vi "Abbreviate TDMS Group Channel.vi"(9 "Channel":string, 10 "Group":string, 11 "File Path Control":path) -> (2 "Cluster":T1, 3 "Abbreviated":string)   [LabVIEW 2019]
uses:
  File_Group_Chan_Abbr.ctl
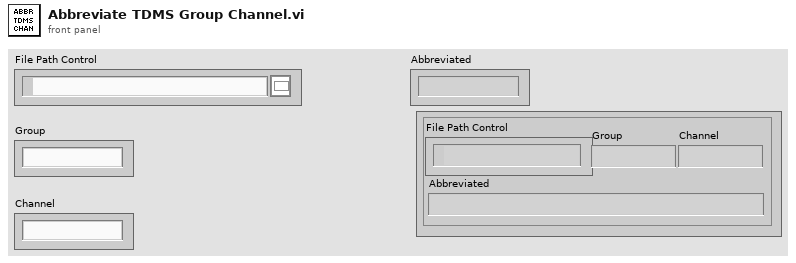
[diagram p1: front panel]
types:
  T1 = typedef "File_Group_Chan_Abbr.ctl" = cluster{"File Path Control":path, "Group":string, "Channel":string, "Abbreviated":string}
  T2 = cluster{"File Path Control":path, "Group":string, "Channel":string, string}
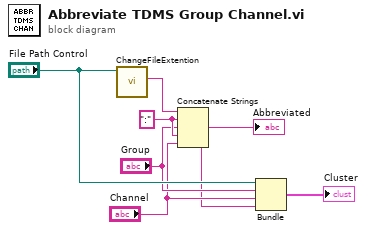
[diagram p0: block diagram]
diagram:
  w6 = ":"
  n1 = call "ChangeFileExtention.vi"("File Path"="File Path Control") -> ("Filename without extension"=w7:string)  [unwired: 5 in, 5 out]
  n2 = Concatenate Strings(w7, w6, "Group", w6, "Channel") -> (w1:string)
  "Abbreviated" <- w1
  n3 = Bundle("File Path Control"="File Path Control", "Group"="Group", "Channel"="Channel", w1) -> (→"Cluster":T2)  [unwired: 1 in]
